vi "openbci_reset_hw_32bit.vi"(8 "error in (no error)":errorcluster, 11 "OBCI dev in":T1={"COM port"="", "n_ch (8)"=enum."8 Channels", "delay_tx"=50}) -> (0 "error out":errorcluster, 3 "OBCI dev out":T1={"COM port"="", "n_ch (8)"=enum."8 Channels", "delay_tx"=50})   [LabVIEW 2013]
doc: "OpenBCI to reset hardware in case of 32bit board"
uses:
  Control Def/openbci_device.ctl
  Control Def/channel_count.ctl
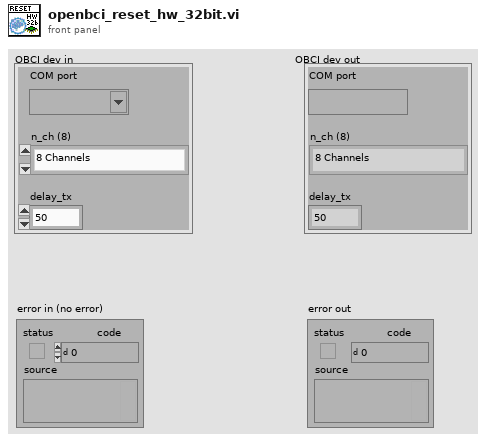
[diagram p1: front panel]
types:
  T1 = typedef "openbci_device.ctl" = cluster{"COM port":refnum<visa-resource-name>, "n_ch (8)":T2, "delay_tx":u32}
  T2 = typedef "channel_count.ctl" = enum16{"8 Channels", "16 Channels"}
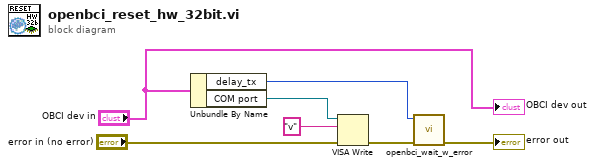
[diagram p0: block diagram]
diagram:
  n1 = Unbundle By Name("OBCI dev in") -> ("delay_tx"=w1:u32, "COM port"=w5:refnum<visa-resource-name>)
  n2 = VISA Write(VISA resource name=w5, write buffer="v", error in (no error)="error in (no error)") -> (error out=w2:errorcluster)  [unwired: 2 out]
  n3 = call "openbci_wait_w_error.vi"("error in (no error)"=w2, "milliseconds to wait"=w1) -> ("error out"=→"error out":errorcluster)  [unwired: 9 in]
  "OBCI dev out" <- "OBCI dev in"
